vi "ProduceGraphFromDropletDbs.vi"(8 "error in (no error)":errorcluster, 10 "Bin Size (Deg)":dbl=0.2, 11 "Droplets Freeze Information":T1=[{"FreezeTemperature"=-34.0, "FreezeFileInformation"="E:\\LINKAM Measurements_Naama\\20150105\\DDWrecycle2-05_01_2015-12_16_42.avi", "Diameter (microns)"=14.614017942303876}, {"FreezeTemperature"=-32.0, "FreezeFileInformation"="E:\\LINKAM Measurements_Naama\\20150105\\DDWrecycle2-05_01_2015-12_16_42.avi", "Diameter (microns)"=10.842816}, {"FreezeTemperature"=-32.0, "FreezeFileInformation"="E:\\LINKAM Measurements_Naama\\20150105\\DDWrecycle2-05_01_2015-12_16_42.avi", "Diameter (microns)"=10.842816}, {"FreezeTemperature"=-32.0, "FreezeFileInformation"="E:\\LINKAM Measurements_Naama\\20150105\\DDWrecycle2-05_01_2015-12_16_42.avi", "Diameter (microns)"=12.198167999999999}, {"FreezeTemperature"=-32.0, "FreezeFileInformation"="E:\\LINKAM Measurements_Naama\\20150105\\DDWrecycle2-05_01_2015-12_16_42.avi", "Diameter (microns)"=12.198167999999999}, {"FreezeTemperature"=-32.0, "FreezeFileInformation"="E:\\LINKAM Measurements_Naama\\20150105\\DDWrecycle2-05_01_2015-12_16_42.avi", "Diameter (microns)"=12.198167999999999}, {"FreezeTemperature"=-32.0, "FreezeFileInformation"="E:\\LINKAM Measurements_Naama\\20150105\\DDWrecycle2-05_01_2015-12_16_42.avi", "Diameter (microns)"=12.198167999999999}, {"FreezeTemperature"=-31.6, "FreezeFileInformation"="E:\\LINKAM Measurements_Naama\\20150105\\DDWrecycle2-05_01_2015-12_16_42.avi", "Diameter (microns)"=12.198167999999999}, {"FreezeTemperature"=-31.0, "FreezeFileInformation"="E:\\LINKAM Measurements_Naama\\20150105\\DDWrecycle2-05_01_2015-12_16_42.avi", "Diameter (microns)"=10.812096467565441}, {"FreezeTemperature"=-31.0, "FreezeFileInformation"="E:\\LINKAM Measurements_Naama\\20150105\\DDWrecycle2-05_01_2015-12_16_42.avi", "Diameter (microns)"=12.294215068392734}, {"FreezeTemperature"=-30.2, "FreezeFileInformation"="E:\\LINKAM Measurements_Naama\\20150105\\DDWrecycle2-05_01_2015-12_16_42.avi", "Diameter (microns)"=13.553519999999999}, {"FreezeTemperature"=-30.2, "FreezeFileInformation"="E:\\LINKAM Measurements_Naama\\20150105\\DDWrecycle2-05_01_2015-12_16_42.avi", "Diameter (microns)"=18.974928}, {"FreezeTemperature"=-30.0, "FreezeFileInformation"="E:\\LINKAM Measurements_Naama\\20150105\\DDWrecycle2-05_01_2015-12_16_42.avi", "Diameter (microns)"=10.384452587272401}, {"FreezeTemperature"=-30.0, "FreezeFileInformation"="E:\\LINKAM Measurements_Naama\\20150105\\DDWrecycle2-05_01_2015-12_16_42.avi", "Diameter (microns)"=10.842816}, {"FreezeTemperature"=-30.0, "FreezeFileInformation"="E:\\LINKAM Measurements_Naama\\20150105\\DDWrecycle2-05_01_2015-12_16_42.avi", "Diameter (microns)"=10.842816}, {"FreezeTemperature"=-30.0, "FreezeFileInformation"="E:\\LINKAM Measurements_Naama\\20150105\\DDWrecycle2-05_01_2015-12_16_42.avi", "Diameter (microns)"=11.645510520165375}, {"FreezeTemperature"=-30.0, "FreezeFileInformation"="E:\\LINKAM Measurements_Naama\\20150105\\DDWrecycle2-05_01_2015-12_16_42.avi", "Diameter (microns)"=21.991369692088856}]) -> (0 "error out":errorcluster, 1 "T50 (Median)":dbl=-30.9975, 2 "NoOfDroplets":i32=17, 3 "Normalized number of Droplets vs. Temperature":cluster{"Ramp Pattern":dbl[], dbl[]}(graph), 4 "T10":dbl=-29.9934, 5 "Normalized number of Droplets vs. Temperature 2":cluster{dbl[], dbl[]}(graph), 6 "Normalized number of Droplets vs. Temperature All Data":cluster{dbl[], dbl[]}(graph))   [LabVIEW 2013]
doc: "Use this template to build a VI to use as a subVI."
uses:
  TypeDef/MultipleFileData.ctl
  <vilib>/Analysis/NI_AALPro.lvlib
  <vilib>/Analysis/NI_AALBase.lvlib
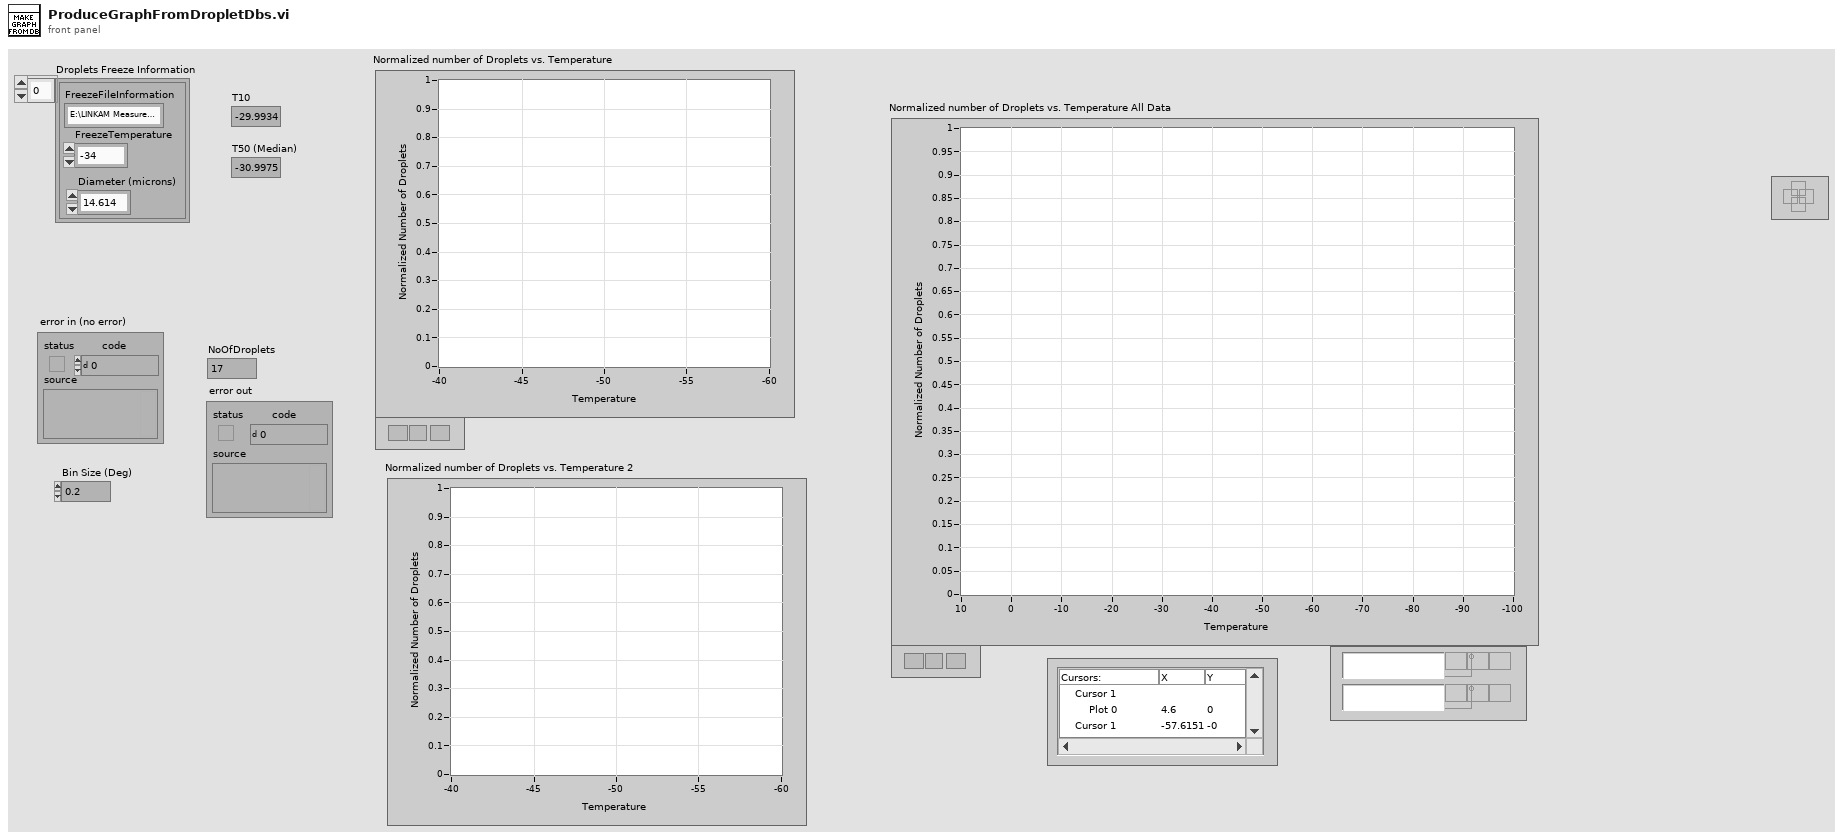
[diagram p1: front panel]
types:
  T1 = typedef "MultipleFileData.ctl" = cluster{"FreezeTemperature":dbl, "FreezeFileInformation":string, "Diameter (microns)":dbl}[]
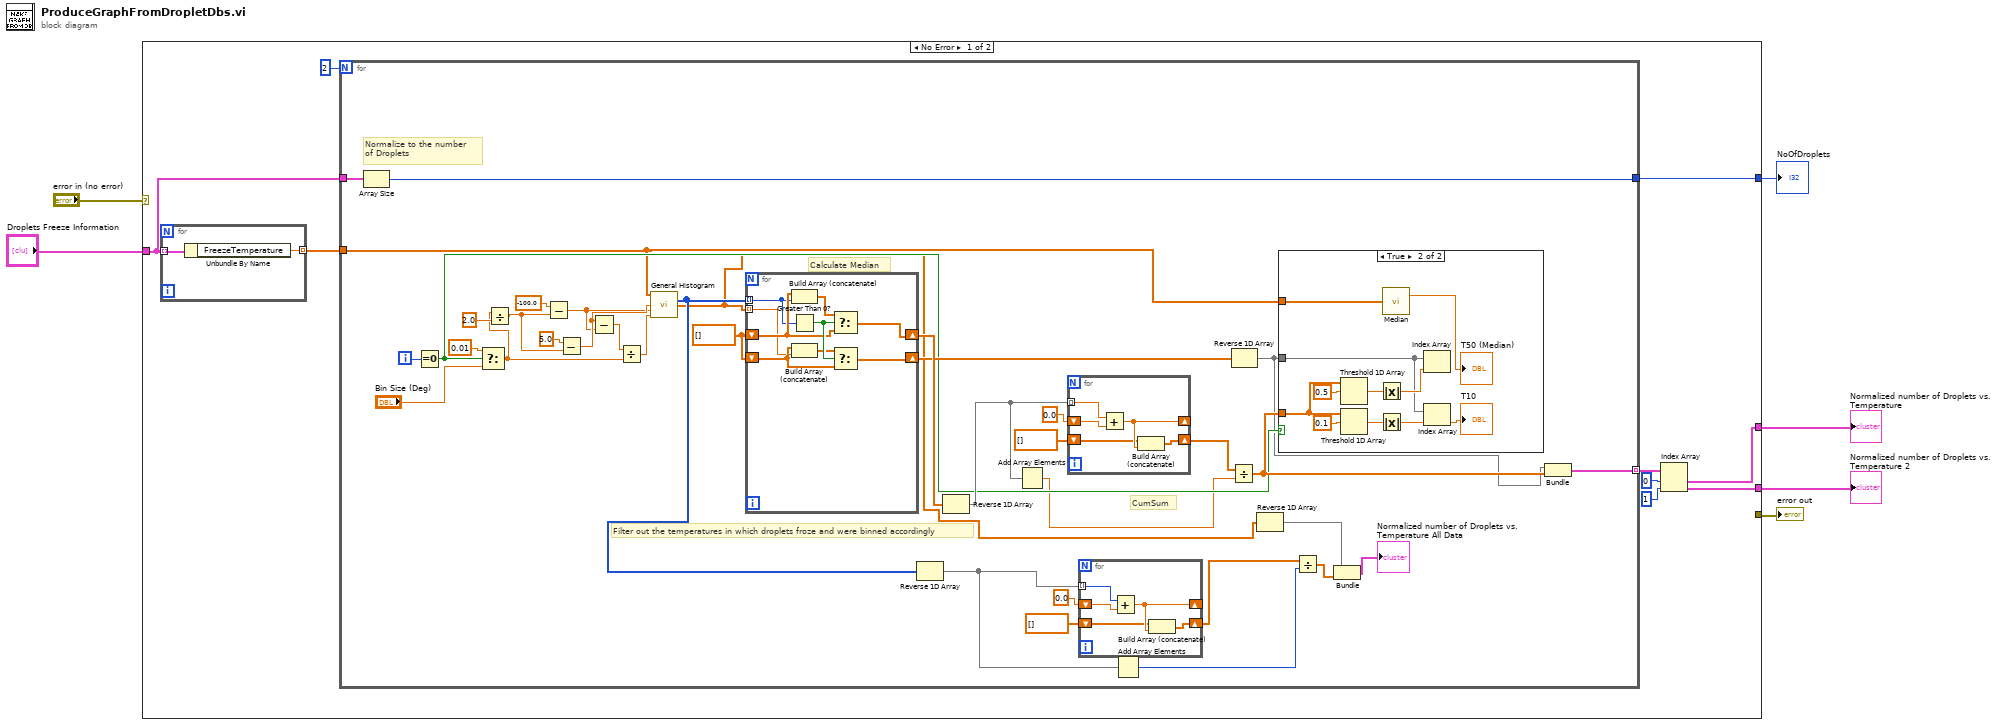
[diagram p0: block diagram]
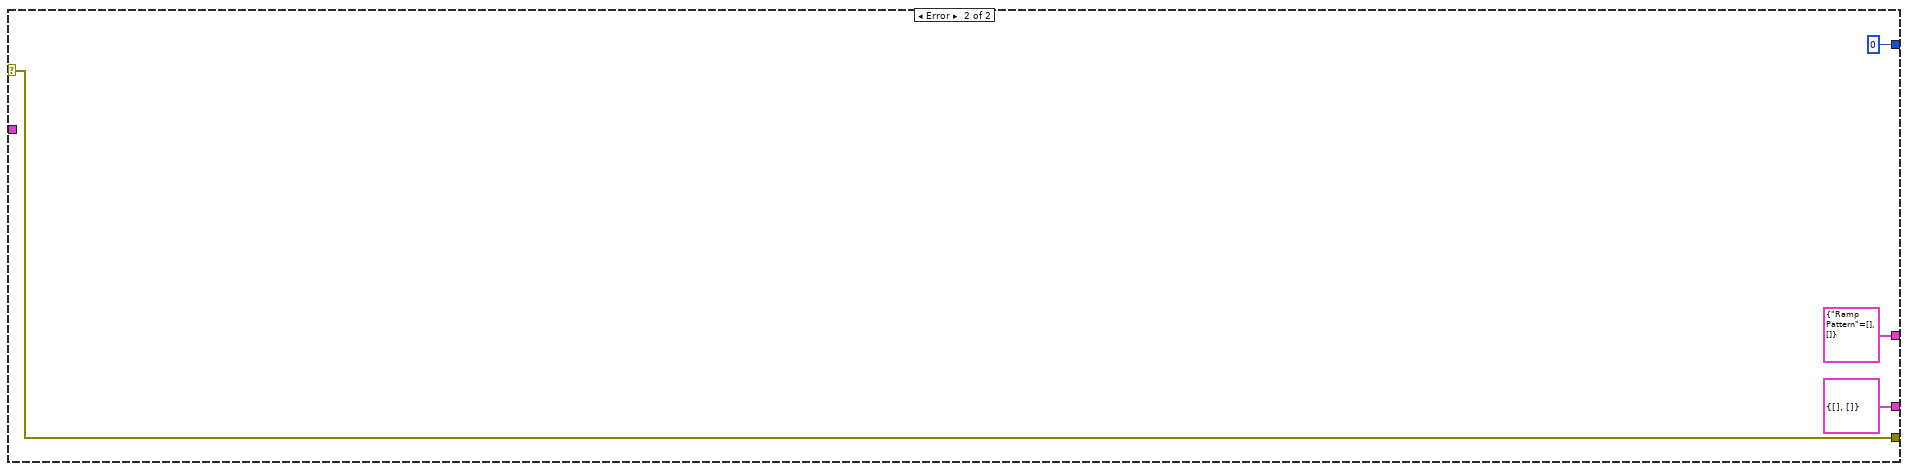
[diagram p3: hidden frame]
diagram:
  n1 = case shown="No Error" "error in (no error)" {
    selector: "error in (no error)" -> [_ w88]
    tunnel: [_ w88] -> w5
    tunnel: "Droplets Freeze Information" -> [w15 _]
    tunnel: [w8 cluster{"Ramp Pattern":dbl[], dbl[]} {"Ramp Pattern"=[], []}] -> w3
    tunnel: [w14 0] -> w2
    tunnel: [w7 cluster{dbl[], dbl[]} {[], []}] -> w1
    frame No Error {
      n2 = for {
        tunnel: w15 -> [w84] mode=indexing
        tunnel: [w83] -> w13 mode=indexing
        n3 = Unbundle By Name(w84) -> ("FreezeTemperature"=w83:dbl)
      }
      n4 = for {
        N: 2 -> [_]
        tunnel: w15 -> [w52]
        tunnel: [w51] -> w14
        tunnel: w13 -> [w16]
        tunnel: [w47] -> w9 mode=indexing
        i -> [w42]
        w50 = dbl[] []
        # "CumSum"
        # "Filter out the temperatures in which droplets froze and were binned accordingly"
        # "Calculate Median"
        # "Normalize to the number \nof Droplets"
        n5 = Array Size(array=w52) -> (size(s)=w51:i32)
        n6 = Equal To 0?(x=w42) -> (x = 0?=w39:bool)
        n7 = Select(t=0.01, s=w39, f="Bin Size (Deg)") -> (s? t:f=w31:dbl)
        n8 = Divide(x=w31, y=2.0) -> (x/y=w30:dbl)
        n9 = Subtract(x=-100.0 ("min"), y=w30) -> (x-y=w33:dbl)
        n10 = Subtract(x=5.0 ("max"), y=w30) -> (x-y=w35:dbl)
        n11 = Subtract(x=w35, y=w33) -> (x-y=w43:dbl)
        n12 = Divide(x=w43, y=w31) -> (x/y=w38:dbl)
        n13 = call <vilib>:"General Histogram.vi"("X"=w16, "max"=w35, "min"=w33, "# bins"=w38) -> ("Histogram"=w18:i32[], "Axis"=w17:dbl[])  [unwired: 7 in, 3 out]
        n14 = for {
          tunnel: w18 -> [w80] mode=indexing
          tunnel: w17 -> [w76] mode=indexing
          shift-right: [w79] -> w46
          shift-left: w50 -> [w81]
          shift-right: [w78] -> w44
          shift-left: w50 -> [w77]
          n15 = Build Array (concatenate)(w81, w80) -> (w74:dbl[])
          n16 = Greater Than 0?(x=w80) -> (x > 0?=w82:bool)
          n17 = Build Array (concatenate)(w77, w76) -> (w75:dbl[])
          n18 = Select(t=w74, s=w82, f=w81) -> (s? t:f=w79:dbl[])
          n19 = Select(t=w75, s=w82, f=w77) -> (s? t:f=w78:dbl[])
        }
        n20 = Reverse 1D Array(array=w18) -> (reversed array=w20:i32[])
        n21 = Reverse 1D Array(array=w46) -> (reversed array=w45:dbl[])
        n22 = Add Array Elements(numeric array=w45) -> (sum=w28:dbl)
        n23 = for {
          tunnel: w45 -> [w70] mode=indexing
          shift-right: [w73] -> w29
          shift-left: dbl[] [] -> [w71]
          shift-right: [w72] -> _
          shift-left: 0.0 -> [w69]
          n24 = Add(x=w70, y=w69) -> (x+y=w72:dbl)
          n25 = Build Array (concatenate)(w71, w72) -> (w73:dbl[])
        }
        n26 = for {
          tunnel: w20 -> [w54] mode=indexing
          shift-right: [w57] -> w23
          shift-left: dbl[] [] -> [w55]
          shift-right: [w56] -> _
          shift-left: 0.0 -> [w53]
          n27 = Add(x=w54, y=w53) -> (x+y=w56:dbl)
          n28 = Build Array (concatenate)(w55, w56) -> (w57:dbl[])
        }
        n29 = Add Array Elements(numeric array=w20) -> (sum=w22:i32)
        n30 = Divide(x=w29, y=w28) -> (x/y=w40:dbl[])
        n31 = Reverse 1D Array(array=w44) -> (reversed array=w26:dbl[])
        n32 = Reverse 1D Array(array=w17) -> (reversed array=w19:dbl[])
        n33 = case shown="True" w39 {
          tunnel: w26 -> [_ w62]
          tunnel: w40 -> [_ w60]
          tunnel: w16 -> [_ w59]
          frame False {
          }
          frame True {
            n34 = Threshold 1D Array(2:0.5 ("threshold y"), 3:w60) -> (0:w65:dbl)  [unwired: 1 in]
            n35 = Threshold 1D Array(2:0.1 ("threshold y"), 3:w60) -> (0:w66:dbl)  [unwired: 1 in]
            n36 = Absolute Value(x=w65) -> (abs(x)=w63:dbl)
            n37 = Absolute Value(x=w66) -> (abs(x)=w64:dbl)
            n38 = call <vilib>:"Median.vi"("X"=w59) -> ("median"=→"T50 (Median)":dbl)  [unwired: 1 out]
            n39 = Index Array(array=w62, index=w63) -> ()  [unwired: 1 out]
            n40 = Index Array(array=w62, index=w64) -> (element=→"T10":dbl)
          }
        }
        n41 = Divide(x=w23, y=w22) -> (x/y=w27:dbl[])
        n42 = Bundle(w19, w27) -> (→"Normalized number of Droplets vs. Temperature All Data":cluster{dbl[], dbl[]})  [unwired: 1 in]
        n43 = Bundle(w26, w40) -> (w47:cluster{dbl[], dbl[]})  [unwired: 1 in]
      }
      n44 = Index Array(array=w9, index #1=0 ("index"), index #2=1 ("index")) -> (element #1=w8:cluster{dbl[], dbl[]}, element #2=w7:cluster{dbl[], dbl[]})
    }
    frame Error {
    }
  }
  "error out" <- w5
  "Normalized number of Droplets vs. Temperature" <- w3
  "NoOfDroplets" <- w2
  "Normalized number of Droplets vs. Temperature 2" <- w1
